vi "Write.vi"(11 "Test Case In":refnum<class "Test PCANBasic.lvclass">) -> (0 "error out":errorcluster, 3 "Test Case Out":refnum<class "Test PCANBasic.lvclass">)   [LabVIEW 2020, in "Test PCANBasic.lvclass"]
uses:
  Test PCANBasic.lvclass
  Test PCANBasic.lvclass/Test PCANBasic.ctl
  source/PCANBasic.lvlib
  source/PCAN Baud.ctl
  source/TPCANHandle.ctl
  <vilib>/Astemes/LUnit/Test Case.lvclass
  source/PCAN Message types.ctl
  source/PCAN Message.ctl
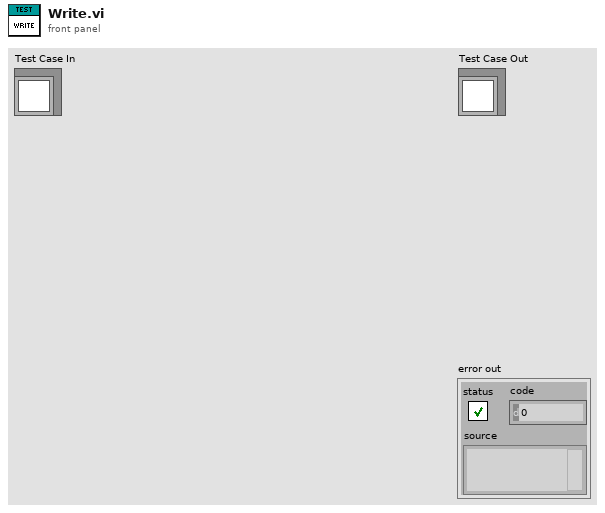
[diagram p1: front panel]
types:
  T1 = cluster{"0":u8, "1":u8, "2":u8, "3":u8, "4":u8, "5":u8, "6":u8, "7":u8}
  T2 = typedef "PCANBasic.lvlib/PCAN Message.ctl" = cluster{"ID":u32, "MSGTYPE":T3, "LEN":u8, "DATA":cluster{"0":u8, "1":u8, "2":u8, "3":u8, "4":u8, "5":u8, "6":u8, "7":u8}}
  T3 = typedef "PCANBasic.lvlib/PCAN Message types.ctl" = u8
  T4 = typedef "PCANBasic.lvlib/TPCANHandle.ctl" = u16
  T5 = typedef "PCANBasic.lvlib/PCAN Baud.ctl" = u16
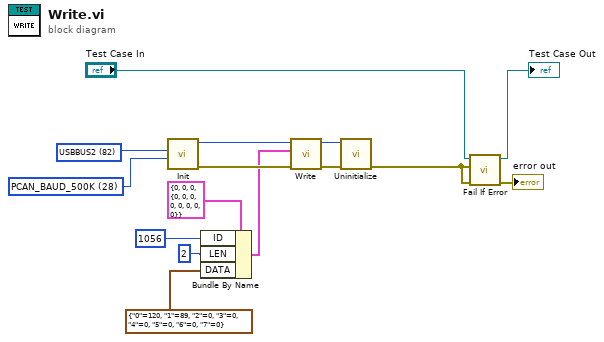
[diagram p0: block diagram]
diagram:
  w11 = T4 82 items=["USBBUS1"=81, "USBBUS2"=82, "USBBUS3"=83, "USBBUS4"=84, "USBBUS5"=85, "USBBUS6"=86, "USBBUS7"=87, "USBBUS8"=88, "USBBUS9"=1289, "USBBUS10"=1290, "USBBUS11"=1291, "USBBUS12"=1292, "USBBUS13"=1293, "USBBUS14"=1294, "USBBUS15"=1295, "USBBUS16"=1296] ("Channel")
  w12 = T5 28 items=["PCAN_BAUD_1M"=20, "PCAN_BAUD_800K"=22, "PCAN_BAUD_500K"=28, "PCAN_BAUD_250K"=284, "PCAN_BAUD_125K"=796, "PCAN_BAUD_100K"=17199, "PCAN_BAUD_95K"=49998, "PCAN_BAUD_83K"=34091, "PCAN_BAUD_50K"=18223, "PCAN_BAUD_47K"=5140, "PCAN_BAUD_33K"=35631, "PCAN_BAUD_20K"=21295, "PCAN_BAUD_10K"=26415, "PCAN_BAUD_5K"=32639] ("Baudrate")
  n1 = call "Init.vi"("Baudrate"=w12, "Channel"=w11) -> ("error out"=w10:errorcluster, "TPCANHandle"=w8:T4)  [unwired: 7 in, 1 out]
  n2 = Bundle By Name(cluster=T2 {"ID"=0, "MSGTYPE"=0, "LEN"=0, "DATA"={"0"=0, "1"=0, "2"=0, "3"=0, "4"=0, "5"=0, "6"=0, "7"=0}} ("PCAN Message"), "ID"=u32 1056, "LEN"=u8 2, "DATA"=T1 {"0"=120, "1"=89, "2"=0, "3"=0, "4"=0, "5"=0, "6"=0, "7"=0}) -> (w2:T2)
  n3 = call "Write.vi"("error in"=w10, "PCAN Message"=w2, "TPCANHandle"=w8) -> ("error out"=w9:errorcluster, "TPCANHandle"=w7:T4)  [unwired: 6 in, 1 out]
  n4 = call "Uninitialize.vi"("error in"=w9, "TPCANHandle"=w7) -> ("error out"=w1:errorcluster)  [unwired: 8 in, 1 out]
  n5 = call <vilib>:"Fail If Error.vi"("error in (no error)"=w1, "Assert error"=w1, "LUnit Test Case In"="Test Case In") -> ("error out"=→"error out":errorcluster, "LUnit Test Case Out"=→"Test Case Out":refnum<class "Test PCANBasic.lvclass">)  [unwired: 7 in]
